vi "Rmv Empt Arr_1D Str.vi"(7 "0번 공란삽입(F)":bool, 8 "error in (no error)":errorcluster caption="에러 입력(에러 없음)", 11 "Data in":string[](array[string])) -> (0 "error out":errorcluster caption="에러 출력", 3 "Data out":string[](array[string]))   [LabVIEW 2020]
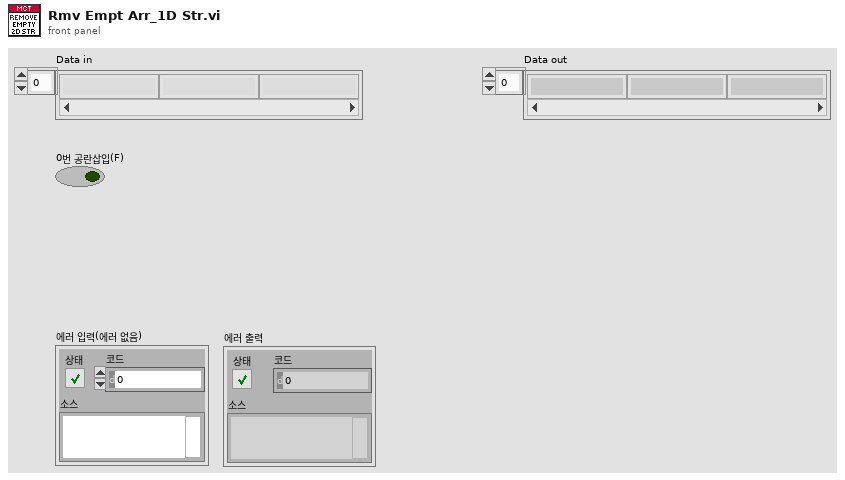
[diagram p1: front panel]
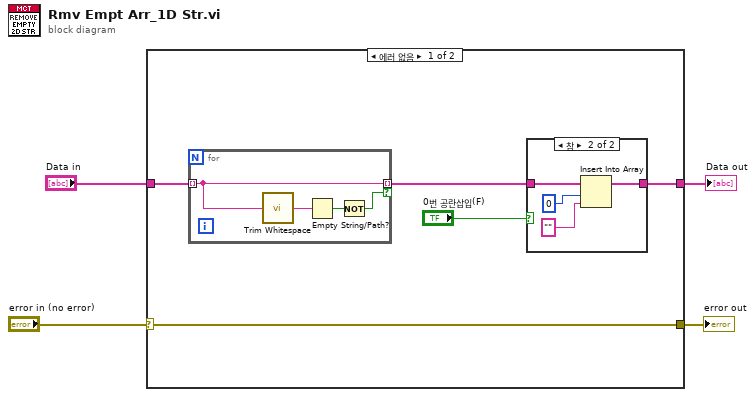
[diagram p0: block diagram]
diagram:
  n1 = case shown="에러 없음" "error in (no error)" {
    selector: "error in (no error)" -> [w8 w20]
    tunnel: "Data in" -> [w9 w19]
    tunnel: [w6 w19] -> w3
    tunnel: [w8 w20] -> w1
    frame No Error {
      n2 = for {
        tunnel: w9 -> [w17] mode=indexing
        tunnel: [w17] -> w7 mode=indexing if=w15
        n3 = call <vilib>:"Trim Whitespace.vi"("string"=w17) -> ("trimmed string"=w18:string)  [unwired: 1 in]
        n4 = Empty String/Path?(string/path=w18) -> (empty?=w16:bool)
        n5 = Not(x=w16) -> (.not. x?=w15:bool)
      }
      n6 = case shown="참" "0번 공란삽입(F)" {
        tunnel: w7 -> [w10 w14]
        tunnel: [w10 w13] -> w6
        frame False {
        }
        frame True {
          n7 = Insert Into Array(array=w14, index=0 ("인덱스"), new element="" ("새 원소/부분배열")) -> (w13:string[])
        }
      }
    }
    frame Error {
    }
  }
  "Data out" <- w3
  "error out" <- w1
